vi "Receive.vi"(6 "Timeout":T1={"mode"=enum."Relative", "deadline (ms)"=30000}, 8 "error in (no error)":errorcluster, 9 "request id":u32, 10 "session in":refnum<class "Session.lvclass">, 11 "command in":refnum<class "SSH_FXP_RMDIR.lvclass">) -> (0 "error out":errorcluster, 1 "unused":i32, 2 "session out":refnum<class "Session.lvclass">, 3 "command out":refnum<class "SSH_FXP_RMDIR.lvclass">)   [LabVIEW 2020, in "NI_SFTP.lvlib" / "SSH_FXP_RMDIR.lvclass"]
uses:
  <vilib>/net/SFTP/API/Support/Command/SSH_FXP_RMDIR/SSH_FXP_RMDIR.lvclass
  <vilib>/net/SFTP/Session/Session.lvclass
  <vilib>/Utility/Deadline/Deadline.ctl
  <vilib>/Utility/Deadline/Mode.ctl
  <vilib>/net/SFTP/NI_SFTP.lvlib
  <vilib>/Utility/Deadline/NI_Deadline.lvlib
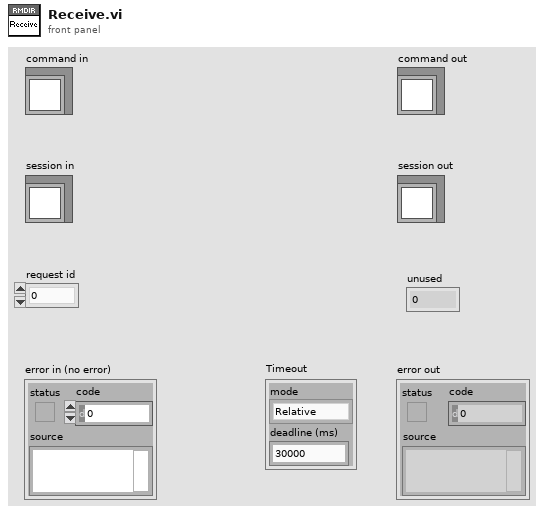
[diagram p1: front panel]
types:
  T1 = typedef "NI_Deadline.lvlib/Deadline.ctl" = cluster{"mode":T2, "deadline (ms)":u32}
  T2 = typedef "NI_Deadline.lvlib/Mode.ctl" = enum16{"Relative", "Use deadline", "Wait forever", "Nonblocking", "N/A"}
  T3 = typedef "NI_SFTP.lvlib/Low Level Connection.lvclass/Packet.ctl" = cluster{"Type":T4, "payload":u8[]}
  T4 = typedef "NI_SFTP.lvlib/Low Level Connection.lvclass/Packet Type.ctl" = enum16{"SSH_FXP_TYPE_000", "SSH_FXP_INIT", "SSH_FXP_VERSION", "SSH_FXP_OPEN", "SSH_FXP_CLOSE", "SSH_FXP_READ", "SSH_FXP_WRITE", "SSH_FXP_LSTAT", "SSH_FXP_FSTAT", "SSH_FXP_SETSTAT", "SSH_FXP_FSETSTAT", "SSH_FXP_OPENDIR", "SSH_FXP_READDIR", "SSH_FXP_REMOVE", "SSH_FXP_MKDIR", "SSH_FXP_RMDIR", "SSH_FXP_REALPATH", "SSH_FXP_STAT", "SSH_FXP_RENAME", "SSH_FXP_READLINK", "SSH_FXP_SYMLINK", "SSH_FXP_LINK", "SSH_FXP_BLOCK", "SSH_FXP_UNBLOCK", "SSH_FXP_TYPE_024", "SSH_FXP_TYPE_025", "SSH_FXP_TYPE_026", "SSH_FXP_TYPE_027", "SSH_FXP_TYPE_028", "SSH_FXP_TYPE_029", "SSH_FXP_TYPE_030", "SSH_FXP_TYPE_031", "SSH_FXP_TYPE_032", "SSH_FXP_TYPE_033", "SSH_FXP_TYPE_034", "SSH_FXP_TYPE_035", "SSH_FXP_TYPE_036", "SSH_FXP_TYPE_037", "SSH_FXP_TYPE_038", "SSH_FXP_TYPE_039", "SSH_FXP_TYPE_040", "SSH_FXP_TYPE_041", "SSH_FXP_TYPE_042", "SSH_FXP_TYPE_043", "SSH_FXP_TYPE_044", "SSH_FXP_TYPE_045", "SSH_FXP_TYPE_046", "SSH_FXP_TYPE_047", "SSH_FXP_TYPE_048", "SSH_FXP_TYPE_049", "SSH_FXP_TYPE_050", "SSH_FXP_TYPE_051", "SSH_FXP_TYPE_052", "SSH_FXP_TYPE_053", "SSH_FXP_TYPE_054", "SSH_FXP_TYPE_055", "SSH_FXP_TYPE_056", "SSH_FXP_TYPE_057", "SSH_FXP_TYPE_058", "SSH_FXP_TYPE_059", "SSH_FXP_TYPE_060", "SSH_FXP_TYPE_061", "SSH_FXP_TYPE_062", "SSH_FXP_TYPE_063", "SSH_FXP_TYPE_064", "SSH_FXP_TYPE_065", "SSH_FXP_TYPE_066", "SSH_FXP_TYPE_067", "SSH_FXP_TYPE_068", "SSH_FXP_TYPE_069", "SSH_FXP_TYPE_070", "SSH_FXP_TYPE_071", "SSH_FXP_TYPE_072", "SSH_FXP_TYPE_073", "SSH_FXP_TYPE_074", "SSH_FXP_TYPE_075", "SSH_FXP_TYPE_076", "SSH_FXP_TYPE_077", "SSH_FXP_TYPE_078", "SSH_FXP_TYPE_079", "SSH_FXP_TYPE_080", "SSH_FXP_TYPE_081", "SSH_FXP_TYPE_082", "SSH_FXP_TYPE_083", "SSH_FXP_TYPE_084", "SSH_FXP_TYPE_085", "SSH_FXP_TYPE_086", "SSH_FXP_TYPE_087", "SSH_FXP_TYPE_088", "SSH_FXP_TYPE_089", "SSH_FXP_TYPE_090", "SSH_FXP_TYPE_091", "SSH_FXP_TYPE_092", "SSH_FXP_TYPE_093", "SSH_FXP_TYPE_094", "SSH_FXP_TYPE_095", "SSH_FXP_TYPE_096", "SSH_FXP_TYPE_097", "SSH_FXP_TYPE_098", "SSH_FXP_TYPE_099", "SSH_FXP_TYPE_100", "SSH_FXP_STATUS", "SSH_FXP_HANDLE", "SSH_FXP_DATA", "SSH_FXP_NAME", "SSH_FXP_ATTRS", "SSH_FXP_TYPE_106", "SSH_FXP_TYPE_107", "SSH_FXP_TYPE_108", "SSH_FXP_TYPE_109", "SSH_FXP_TYPE_110", "SSH_FXP_TYPE_111", "SSH_FXP_TYPE_112", "SSH_FXP_TYPE_113", "SSH_FXP_TYPE_114", "SSH_FXP_TYPE_115", "SSH_FXP_TYPE_116", "SSH_FXP_TYPE_117", "SSH_FXP_TYPE_118", "SSH_FXP_TYPE_119", "SSH_FXP_TYPE_120", "SSH_FXP_TYPE_121", "SSH_FXP_TYPE_122", "SSH_FXP_TYPE_123", "SSH_FXP_TYPE_124", "SSH_FXP_TYPE_125", "SSH_FXP_TYPE_126", "SSH_FXP_TYPE_127", "SSH_FXP_TYPE_128", "SSH_FXP_TYPE_129", "SSH_FXP_TYPE_130", "SSH_FXP_TYPE_131", "SSH_FXP_TYPE_132", "SSH_FXP_TYPE_133", "SSH_FXP_TYPE_134", "SSH_FXP_TYPE_135", "SSH_FXP_TYPE_136", "SSH_FXP_TYPE_137", "SSH_FXP_TYPE_138", "SSH_FXP_TYPE_139", "SSH_FXP_TYPE_140", "SSH_FXP_TYPE_141", "SSH_FXP_TYPE_142", "SSH_FXP_TYPE_143", "SSH_FXP_TYPE_144", "SSH_FXP_TYPE_145", "SSH_FXP_TYPE_146", "SSH_FXP_TYPE_147", "SSH_FXP_TYPE_148", "SSH_FXP_TYPE_149", "SSH_FXP_TYPE_150", "SSH_FXP_TYPE_151", "SSH_FXP_TYPE_152", "SSH_FXP_TYPE_153", "SSH_FXP_TYPE_154", "SSH_FXP_TYPE_155", "SSH_FXP_TYPE_156", "SSH_FXP_TYPE_157", "SSH_FXP_TYPE_158", "SSH_FXP_TYPE_159", "SSH_FXP_TYPE_160", "SSH_FXP_TYPE_161", "SSH_FXP_TYPE_162", "SSH_FXP_TYPE_163", "SSH_FXP_TYPE_164", "SSH_FXP_TYPE_165", "SSH_FXP_TYPE_166", "SSH_FXP_TYPE_167", "SSH_FXP_TYPE_168", "SSH_FXP_TYPE_169", "SSH_FXP_TYPE_170", "SSH_FXP_TYPE_171", "SSH_FXP_TYPE_172", "SSH_FXP_TYPE_173", "SSH_FXP_TYPE_174", "SSH_FXP_TYPE_175", "SSH_FXP_TYPE_176", "SSH_FXP_TYPE_177", "SSH_FXP_TYPE_178", "SSH_FXP_TYPE_179", "SSH_FXP_TYPE_180", "SSH_FXP_TYPE_181", "SSH_FXP_TYPE_182", "SSH_FXP_TYPE_183", "SSH_FXP_TYPE_184", "SSH_FXP_TYPE_185", "SSH_FXP_TYPE_186", "SSH_FXP_TYPE_187", "SSH_FXP_TYPE_188", "SSH_FXP_TYPE_189", "SSH_FXP_TYPE_190", "SSH_FXP_TYPE_191", "SSH_FXP_TYPE_192", "SSH_FXP_TYPE_193", "SSH_FXP_TYPE_194", "SSH_FXP_TYPE_195", "SSH_FXP_TYPE_196", "SSH_FXP_TYPE_197", "SSH_FXP_TYPE_198", "SSH_FXP_TYPE_199", "SSH_FXP_EXTENDED", "SSH_FXP_EXTENDED_REPLY"}
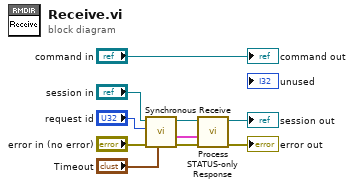
[diagram p0: block diagram]
diagram:
  n1 = call <vilib>:"Synchronous Receive.vi"("Timeout"="Timeout", "error in (no error)"="error in (no error)", "request id"="request id", "session in"="session in") -> ("error out"=w5:errorcluster, "packet"=w2:T3, "session out"=w4:refnum<class "Session.lvclass">)  [unwired: 5 in]
  n2 = call <vilib>:"Process STATUS-only Response.vi"("error in"=w5, "packet"=w2, "session in"=w4) -> ("error out"=→"error out":errorcluster, "session out"=→"session out":refnum<class "Session.lvclass">)  [unwired: 7 in]
  "command out" <- "command in"
